vi "startUp.vi"(8 "error in (no error)":errorcluster, 11 "ScriptEditorV2 in":refnum<class "ScriptEditorV2.lvclass">) -> (0 "error out":errorcluster, 3 "ScriptEditorV2 out":refnum<class "ScriptEditorV2.lvclass">)   [LabVIEW 2009, in "Views.lvlib" / "ScriptEditor.lvlib" / "ScriptEditorV2.lvclass"]
uses:
  ScriptEditorV2.lvclass
  Tools/Scripting/ScriptingEvent/ScriptEventList/ScriptEventList.lvclass
  ScriptEditorV2.lvclass/ScriptEditorV2.ctl
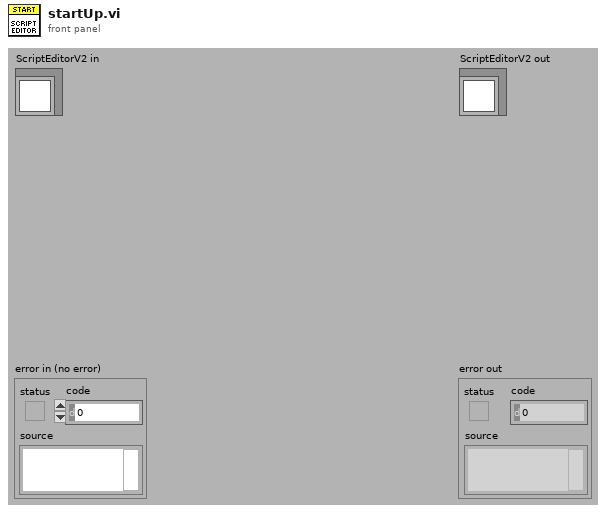
[diagram p1: front panel]
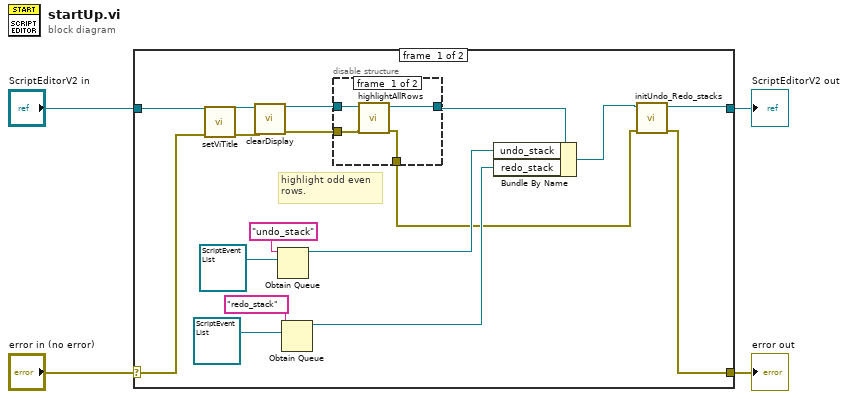
[diagram p0: block diagram]
diagram:
  n1 = case shown="No Error" "error in (no error)" {
    selector: "error in (no error)" -> [w21 w29]
    tunnel: [w5 w29] -> w3
    tunnel: [w7 w28] -> w1
    tunnel: "ScriptEditorV2 in" -> [w20 w28]
    frame #0 {
      # "highlight odd even\nrows."
      n2 = call "setViTitle.vi"("error in (no error)"=w21, "ScriptEditorV2 in"=w20) -> ("error out"=w18:errorcluster, "ScriptEditorV2 out"=w19:refnum<class "ScriptEditorV2.lvclass">)  [unwired: 8 in]
      n3 = call "clearDisplay.vi"("error in (no error)"=w18, "ScriptEditorV2 in"=w19) -> ("error out"=w16:errorcluster, "ScriptEditorV2 out"=w17:refnum<class "ScriptEditorV2.lvclass">)  [unwired: 8 in]
      n4 = Obtain Queue(name (unnamed)="undo_stack", element data type=refnum<class "ScriptEventList.lvclass"> refnum ("ScriptEventList")) -> (queue out=w11:refnum<queue>)  [unwired: 3 in, 2 out]
      n5 = Obtain Queue(name (unnamed)="redo_stack", element data type=refnum<class "ScriptEventList.lvclass"> refnum ("ScriptEventList")) -> (queue out=w10:refnum<queue>)  [unwired: 3 in, 2 out]
      n6 = disable-structure shown="Enabled" {
        disable-tunnel: w17 -> [w25 w26]
        disable-tunnel: [w24 w26] -> w9
        disable-tunnel: w16 -> [w23 w27]
        disable-tunnel: [w22 w27] -> w6
        frame #0 {
          n7 = call "highlightAllRows.vi"("error in (no error)"=w23, "ScriptEditorV2 in"=w25) -> ("error out"=w22:errorcluster, "ScriptEditorV2 out"=w24:refnum<class "ScriptEditorV2.lvclass">)  [unwired: 8 in]
        }
        frame #1 {
        }
      }
      n8 = Bundle By Name(cluster=w9, "undo_stack"=w11, "redo_stack"=w10) -> (w8:refnum<class "ScriptEditorV2.lvclass">)
      n9 = call "initUndo_Redo_stacks.vi"("error in (no error)"=w6, "ScriptEditorV2 in"=w8) -> ("error out"=w5:errorcluster, "ScriptEditorV2 out"=w7:refnum<class "ScriptEditorV2.lvclass">)  [unwired: 8 in]
    }
    frame #1 {
    }
  }
  "error out" <- w3
  "ScriptEditorV2 out" <- w1
